vi "RecipeUpdateSeqLine.vi"(4 "LogClear?":bool, 6 "Seq_Index":i32, 8 "error in (no error)":errorcluster, 9 "Message_Queues":T1, 10 "Recipe_Input":string[][](array[string]), 11 "DeviceSetup":variant[](array[variant])) -> (0 "error out":errorcluster, 3 "DeviceSetup_Update":variant[](array[variant]))   [LabVIEW 2014]
uses:
  02_Controls/Message_Queues.ctl
  02_Controls/Message_Data_Ctl.ctl
  Config_RFSA_Spectrum_Acq.ctl
  Config_RFSA_IQ_Acq.ctl
  Config_RFSA_Vertical.ctl
  Config_RFSG.ctl
  Analysis_Parameters.ctl
panel:
  in  "Standard":T2(ring)
  out "Array":dbl[](array[numeric]) format="%#_6p"
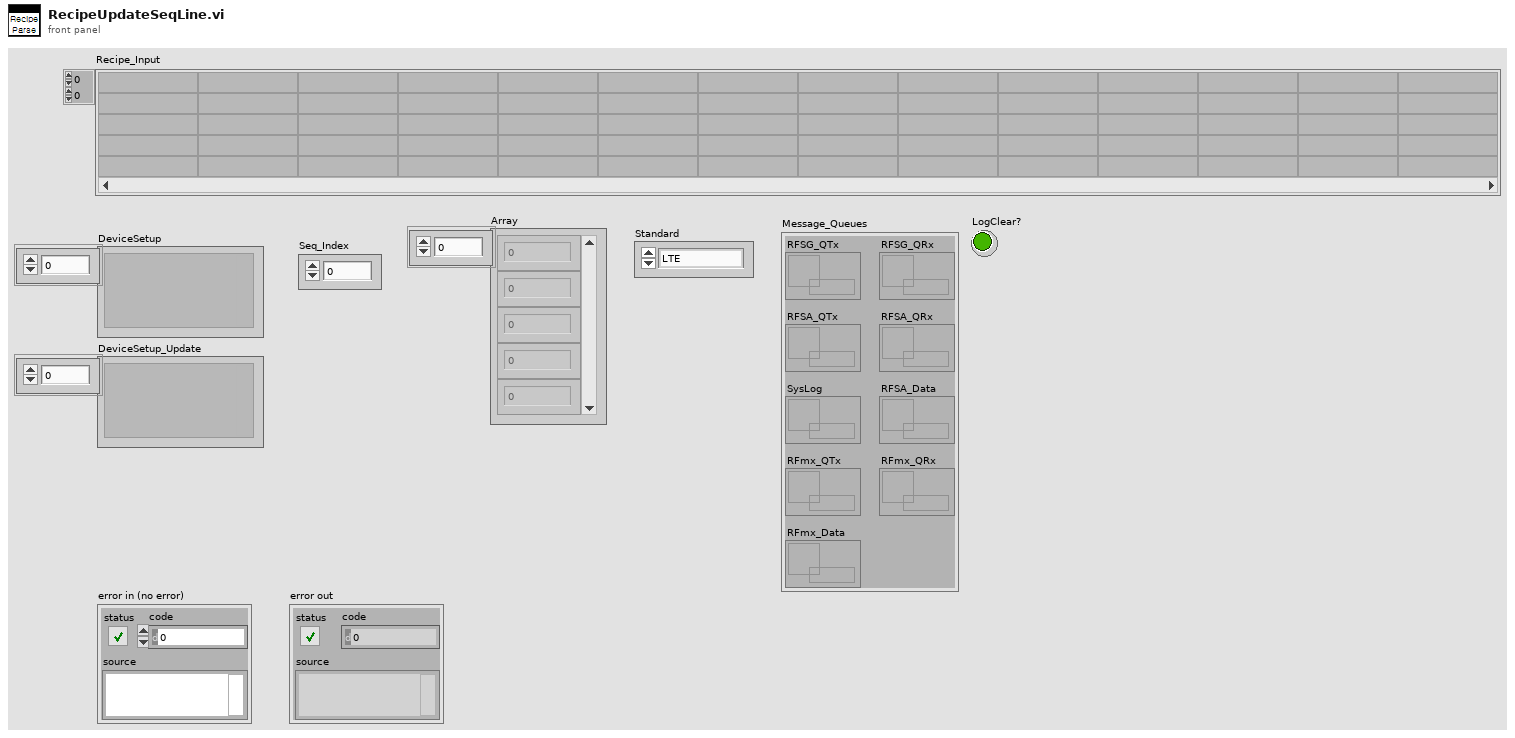
[diagram p1: front panel]
types:
  T1 = typedef "Message_Queues.ctl" = cluster{"RFSG_QTx":refnum<queue>, "RFSG_QRx":refnum<queue>, "RFSA_QTx":refnum<queue>, "RFSA_QRx":refnum<queue>, "SysLog":refnum<queue>, "RFSA_Data":refnum<queue>, "RFmx_QTx":refnum<queue>, "RFmx_QRx":refnum<queue>, "RFmx_Data":refnum<queue>}
  T2 = enum16{"LTE", "WCDMA", "GSM", "EDGE", "CW", "CWM"}
  T3 = typedef "Analysis_Parameters.ctl" = cluster{"carrier frequency":dbl, "IQ rate (S/s)":dbl, "samples per record":i64, "Signal Bandwidth (Hz)":dbl, "Resolution Bandwidth (Hz)":dbl, "Ref ch Bandwidth (Hz)":dbl, "Offset_Freq(Hz)":dbl[], "Integration_Bandwidth(Hz)":dbl[]}
  T4 = typedef "Config_RFSG.ctl" = cluster{"Carrier Frequency":dbl, "RF Power Level (dBm)":dbl, "SG External Gain (dBm)":dbl, "Standard":enum16{"LTE", "WCDMA", "GSM", "EDGE", "CW", "CWM"}}
  T5 = typedef "Config_RFSA_Vertical.ctl" = cluster{"Acquisition Type":i32, "Reference Level (dBm)":dbl, "External Gain (dB)":dbl}
  T6 = typedef "Config_RFSA_IQ_Acq.ctl" = cluster{"carrier frequency":dbl, "IQ rate (S/s)":dbl, "samples per record":i64}
  T7 = typedef "Config_RFSA_Spectrum_Acq.ctl" = cluster{"Resolution Bandwidth (Hz)":dbl, "Start Frequency (Hz)":dbl, "Stop Frequency (Hz)":dbl}
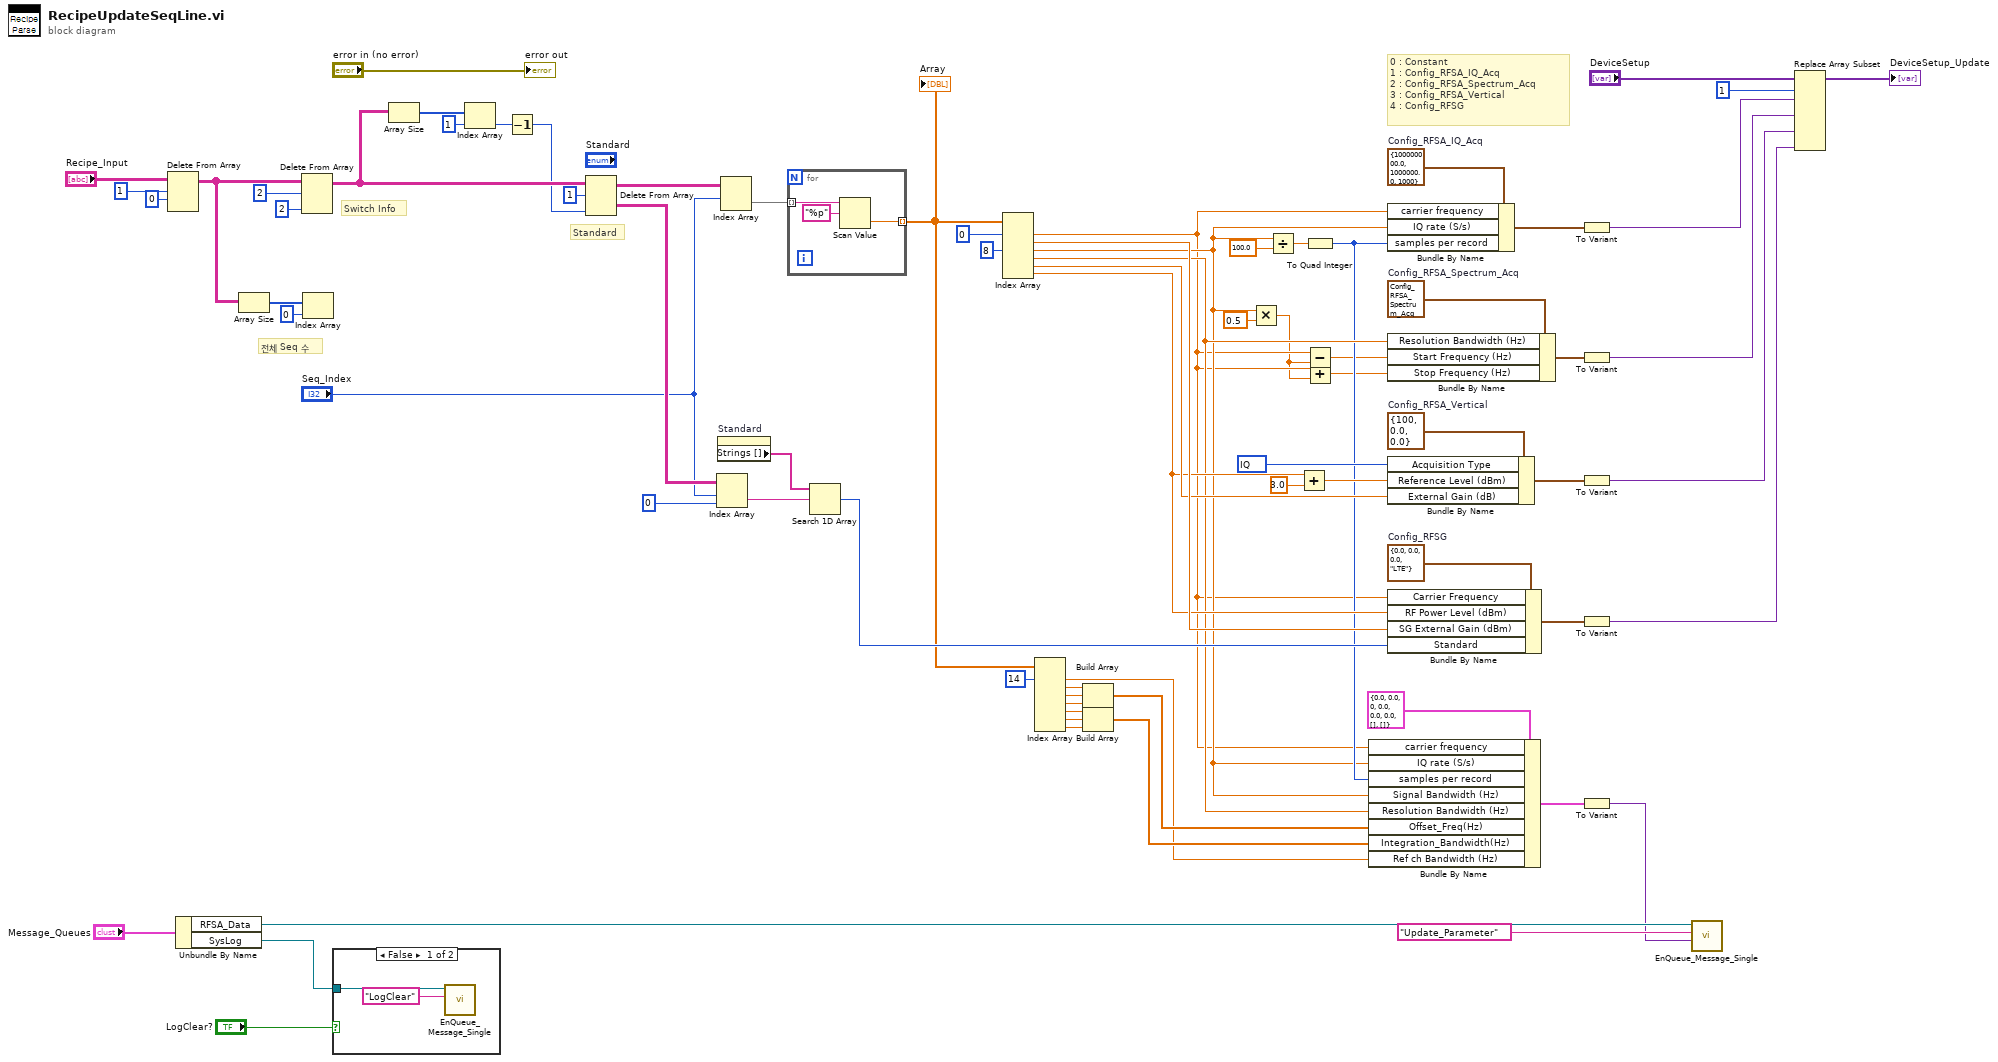
[diagram p0: block diagram]
diagram:
  w59 = T4 {"Carrier Frequency"=0.0, "RF Power Level (dBm)"=0.0, "SG External Gain (dBm)"=0.0, "Standard"=enum."LTE"}  # Config_RFSG
  w53 = 100 items=["IQ"=100, "Spectrum"=101] ("Acquisition Type")
  w56 = T5 {"Acquisition Type"=100, "Reference Level (dBm)"=0.0, "External Gain (dB)"=0.0}  # Config_RFSA_Vertical
  w58 = T6 {"carrier frequency"=100000000.0, "IQ rate (S/s)"=1000000.0, "samples per record"=1000}  # Config_RFSA_IQ_Acq
  w57 = T7 {"Resolution Bandwidth (Hz)"=10000.0, "Start Frequency (Hz)"=90000000.0, "Stop Frequency (Hz)"=110000000.0}  # Config_RFSA_Spectrum_Acq
  # "0 : Constant\n1 : Config_RFSA_IQ_Acq\n2 : Config_RFSA_Spectrum_Acq\n3 : Config_RFSA_Vertical\n4 : Config_RFSG"
  # "Switch Info"
  # "Standard"
  # "전체 Seq 수"
  n1 = Delete From Array(array="Recipe_Input", length=1, index (row)=0) -> (array with subset deleted=w71:string[][])  [unwired: 1 in, 1 out]
  n2 = Unbundle By Name("Message_Queues") -> ("RFSA_Data"=w20:refnum<queue>, "SysLog"=w28:refnum<queue>)
  n3 = Array Size(array=w71) -> (size(s)=w73:i32[])
  n4 = Delete From Array(array=w71, length=2, index (col)=2 ("disabled index (col)")) -> (array with subset deleted=w66:string[][])  [unwired: 1 in, 1 out]
  n5 = Index Array(array=w73, index=0) -> ()  [unwired: 1 out]
  n6 = case shown="False" "LogClear?" {
    tunnel: w28 -> [w77 _]
    frame False {
      n7 = call "EnQueue_Message_Single.vi"("Message"="LogClear", "Message_Queue"=w77) -> ()  [unwired: 8 in, 2 out]
    }
    frame True {
    }
  }
  n8 = Array Size(array=w66) -> (size(s)=w68:i32[])
  n9 = Index Array(array=w68, index=1) -> (element=w65:i32)
  n10 = Decrement(x=w65) -> (x-1=w63:i32)
  n11 = Delete From Array(array=w66, length=1, index (col)=w63) -> (deleted portion=w47:string[][], array with subset deleted=w62:string[][])  [unwired: 1 in]
  n12 = Index Array(array=w47, index (row)="Seq_Index", index (col)=0 ("disabled index (col)")) -> (element=w44:string)
  n13 = property on="Standard" class="Enum (strict)"() -> ("Strings []"=w43:string[])  [unwired: 2 in, 2 out]
  n14 = Index Array(array=w62, index (row)="Seq_Index") -> (element=w61:string[])  [unwired: 1 in]
  n15 = for {
    tunnel: w61 -> [w80] mode=indexing
    tunnel: [w78] -> w24 mode=indexing
    n16 = Scan Value(string=w80, format string="%p") -> (value=w78:dbl)  [unwired: 1 in, 1 out]
  }
  "Array" <- w24
  n17 = Search 1D Array(1D array=w43, element=w44) -> (index of element=w42:i32)  [unwired: 1 in]
  n18 = Index Array(array=w24, index #1=0 ("index"), index #3=8 ("index")) -> (element #1=w4:dbl, element #2=w55:dbl, element #3=w7:dbl, element #4=w25:dbl, element #5=w52:dbl, element #6=w51:dbl)  [unwired: 4 in]
  n19 = Index Array(array=w24, index #1=14 ("index")) -> (element #1=w10:dbl, element #2=w11:dbl, element #3=w12:dbl, element #4=w13:dbl, element #5=w14:dbl, element #6=w15:dbl, element #7=w16:dbl)  [unwired: 6 in]
  n20 = Build Array(w11, w12, w13) -> (w22:dbl[])
  n21 = Build Array(w14, w15, w16) -> (w21:dbl[])
  n22 = Multiply(x=w7, y=0.5) -> (x*y=w3:dbl)
  n23 = Divide(x=w7, y=100.0) -> (x/y=w49:dbl)
  n24 = Add(x=w51, y=3.0) -> (x+y=w9:dbl)
  n25 = To Quad Integer(1:w49) -> (0:w8:i64)
  n26 = Subtract(x=w4, y=w3) -> (x-y=w5:dbl)
  n27 = Add(x=w4, y=w3) -> (x+y=w2:dbl)
  n28 = Bundle By Name(cluster=T3 {"carrier frequency"=0.0, "IQ rate (S/s)"=0.0, "samples per record"=0, "Signal Bandwidth (Hz)"=0.0, "Resolution Bandwidth (Hz)"=0.0, "Ref ch Bandwidth (Hz)"=0.0, "Offset_Freq(Hz)"=[], "Integration_Bandwidth(Hz)"=[]} ("Analysis_Parameters"), "carrier frequency"=w4, "IQ rate (S/s)"=w7, "samples per record"=w8, "Signal Bandwidth (Hz)"=w7, "Resolution Bandwidth (Hz)"=w25, "Offset_Freq(Hz)"=w22, "Integration_Bandwidth(Hz)"=w21, "Ref ch Bandwidth (Hz)"=w10) -> (w18:T3)
  n29 = Bundle By Name(cluster=w58, "carrier frequency"=w4, "IQ rate (S/s)"=w7, "samples per record"=w8) -> (w41:T6)
  n30 = Bundle By Name(cluster=w57, "Resolution Bandwidth (Hz)"=w25, "Start Frequency (Hz)"=w5, "Stop Frequency (Hz)"=w2) -> (w40:T7)
  n31 = Bundle By Name(cluster=w56, "Acquisition Type"=w53, "Reference Level (dBm)"=w9, "External Gain (dB)"=w52) -> (w39:T5)
  n32 = Bundle By Name(cluster=w59, "Carrier Frequency"=w4, "RF Power Level (dBm)"=w51, "SG External Gain (dBm)"=w55, "Standard"=w42) -> (w38:T4)
  n33 = To Variant(anything=w41) -> (Variant=w35:variant)
  n34 = To Variant(anything=w40) -> (Variant=w34:variant)
  n35 = To Variant(anything=w39) -> (Variant=w33:variant)
  n36 = To Variant(anything=w38) -> (Variant=w32:variant)
  n37 = To Variant(anything=w18) -> (Variant=w17:variant)
  n38 = call "EnQueue_Message_Single.vi"("Message Data"=w17, "Message"="Update_Parameter", "Message_Queue"=w20) -> ()  [unwired: 7 in, 2 out]
  n39 = Replace Array Subset(array="DeviceSetup", new element #1=w35, index #1=1 ("index"), new element #2=w34, new element #3=w33, new element #4=w32) -> (→"DeviceSetup_Update":variant[])  [unwired: 3 in]
  "error out" <- "error in (no error)"
